vi "GEN_CulArray.vi"(8 "Max Values":i32, 9 "Data_Cluster":T1) -> (1 "Data_Cluster Out":T1)   [LabVIEW 2021]
uses:
  Data_Cluster.ctl
  Measurement_Cluster.ctl
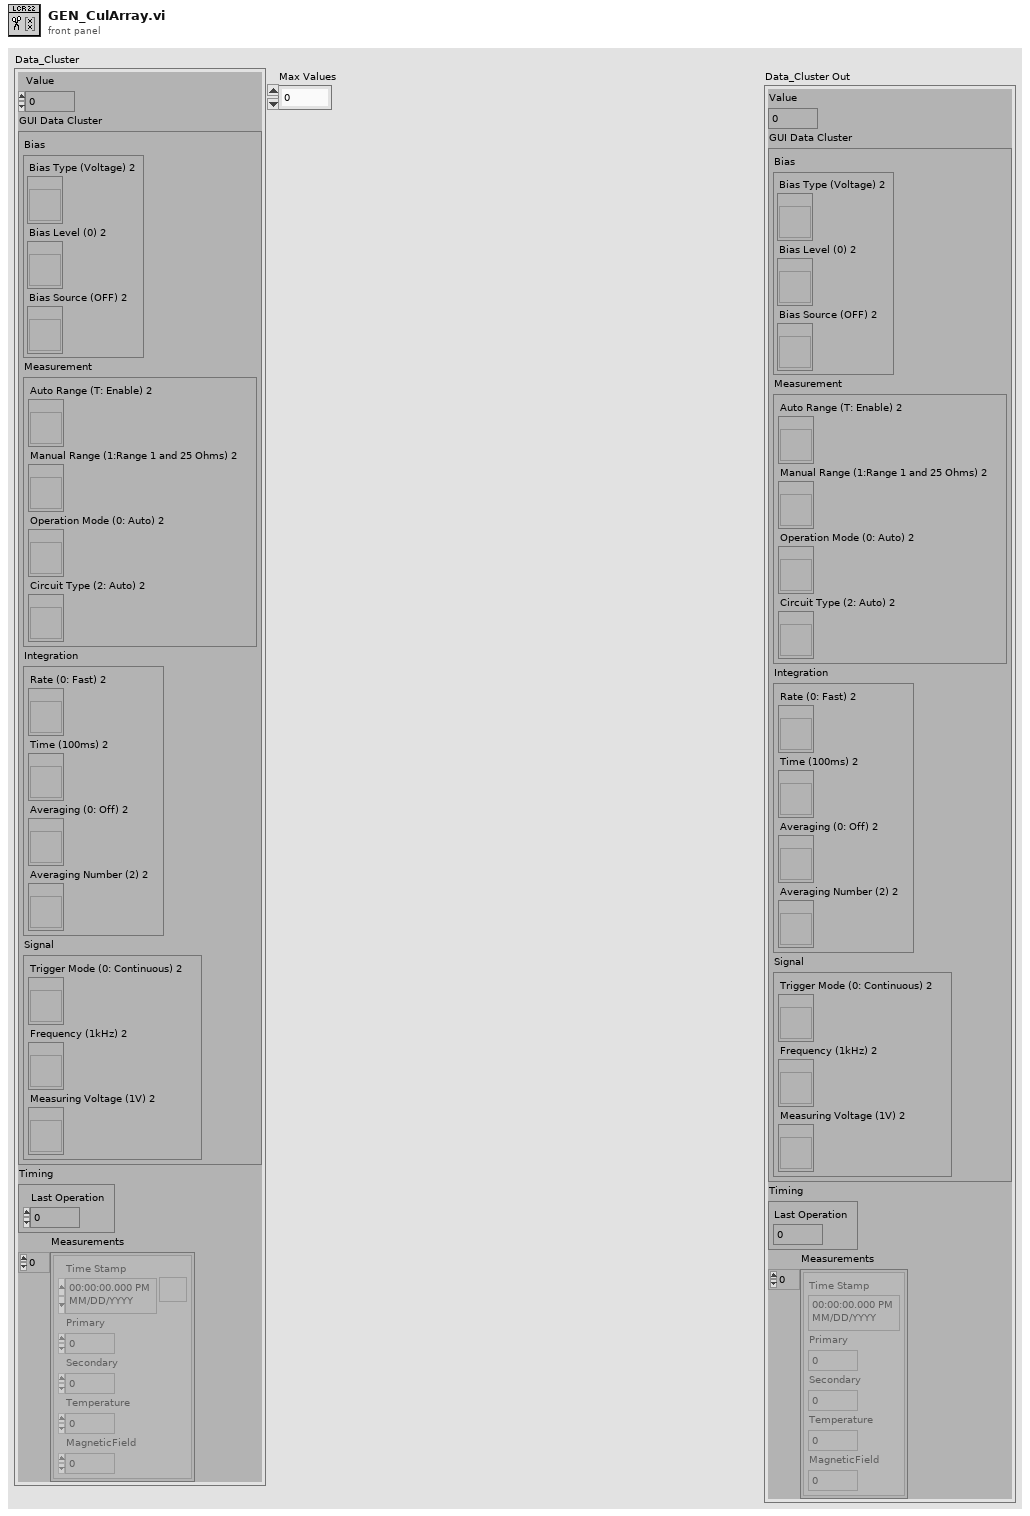
[diagram p1: front panel]
types:
  T1 = typedef "Data_Cluster.ctl" = cluster{"Value":dbl, "GUI Data Cluster":cluster{"Bias":cluster{"Bias Type (Voltage) 2":refnum<vi>, "Bias Level (0) 2":refnum<vi>, "Bias Source (OFF) 2":refnum<vi>}, "Measurement":cluster{"Auto Range (T: Enable) 2":refnum<vi>, "Manual Range (1:Range 1 and 25 Ohms) 2":refnum<vi>, "Operation Mode (0: Auto) 2":refnum<vi>, "Circuit Type (2: Auto) 2":refnum<vi>}, "Integration":cluster{"Rate (0: Fast) 2":refnum<vi>, "Time (100ms) 2":refnum<vi>, "Averaging (0: Off) 2":refnum<vi>, "Averaging Number (2) 2":refnum<vi>}, "Signal":cluster{"Trigger Mode (0: Continuous) 2":refnum<vi>, "Frequency (1kHz) 2":refnum<vi>, "Measuring Voltage (1V) 2":refnum<vi>}}, "Timing":cluster{"Last Operation":dbl}, "Measurements":T2[]}
  T2 = typedef "Measurement_Cluster.ctl" = cluster{"Time Stamp":timestamp, "Primary":dbl, "Secondary":dbl, "Temperature":dbl, "MagneticField":dbl}
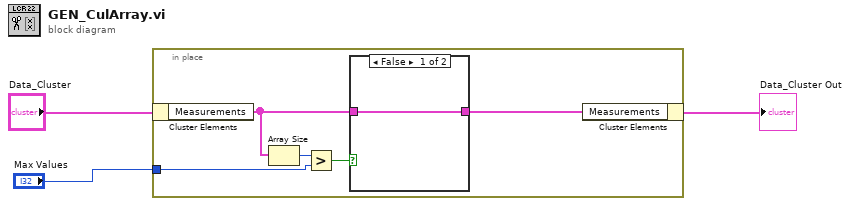
[diagram p0: block diagram]
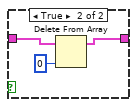
[diagram p2: hidden frame]
diagram:
  n1 = in-place {
    in-place-border: "Max Values" -> [w7]
    n2 = in-place-cluster #1("Data_Cluster") -> ("Measurements"=w5:T2[])
    n3 = Array Size(array=w5) -> (size(s)=w8:i32)
    n4 = Greater?(x=w8, y=w7) -> (0:w6:bool)
    n5 = case shown="False" w6 {
      tunnel: w5 -> [w9 w12]
      tunnel: [w9 w11] -> w4
      frame False {
      }
      frame True {
        n6 = Delete From Array(array=w12, index=0) -> (array with subset deleted=w11:T2[])  [unwired: 1 in, 1 out]
      }
    }
    n7 = in-place-cluster #1("Measurements"=w4) -> (→"Data_Cluster Out":T1)
  }
